vi "roboRIO v1.0 Close RSL.vi"(8 "error in (no error)":errorcluster, 10 "RSL Channel List":T3, 11 "myRIO Ref In":T1) -> (0 "error out":errorcluster)   [LabVIEW 2021]
uses:
  <vilib>/myRIO/Common/Instrument Driver Framework/roboRIO v1.0/RSL/typedefs/RSL Channels List.ctl
  <vilib>/myRIO/Common/Instrument Driver Framework/roboRIO v1.0/RSL/typedefs/RSL Channels Enum.ctl
  <vilib>/myRIO/Common/Instrument Driver Framework/Utilities/typedefs/myRIO v1.0 Reference.ctl
  <vilib>/myRIO/Common/Instrument Driver Framework/Utilities/typedefs/Generic FPGA Reference.ctl
  <vilib>/myRIO/Common/Instrument Driver Framework/roboRIO v1.0/RSL/vis/roboRIO v1.0 Build MUX Configuration RSL.vi
  <vilib>/myRIO/Common/Instrument Driver Framework/roboRIO v1.0/Resource Manager/vis/roboRIO v1.0 Unreserve Channel List.vi
  <vilib>/myRIO/Common/Instrument Driver Framework/roboRIO v1.0/Resource Manager/vis/roboRIO v1.0 Unreserve Channel.vi
  <vilib>/myRIO/Common/Instrument Driver Framework/roboRIO v1.0/Resource Manager/vis/roboRIO v1.0 Build Mutex Name.vi
  <vilib>/myRIO/Common/Instrument Driver Framework/Utilities/vis/Configuration Manager.vi
  <vilib>/myRIO/Common/Instrument Driver Framework/Utilities/vis/IO Manager.vi
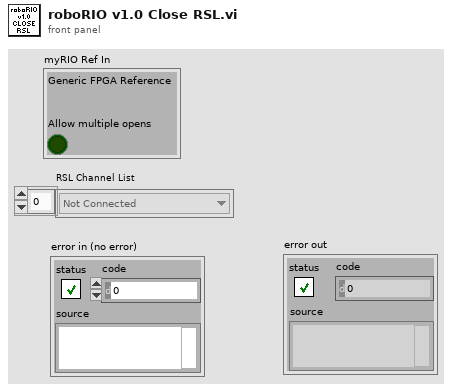
[diagram p1: front panel]
types:
  T1 = typedef "myRIO v1.0 Reference.ctl" = cluster{"Generic FPGA Reference":T2, "Allow multiple opens":bool}
  T2 = typedef "Generic FPGA Reference.ctl" = refnum<k20>
  T3 = typedef "RSL Channels List.ctl" = T4[]
  T4 = typedef "RSL Channels Enum.ctl" = enum16{"Not Connected", "RSL/RSL0"}
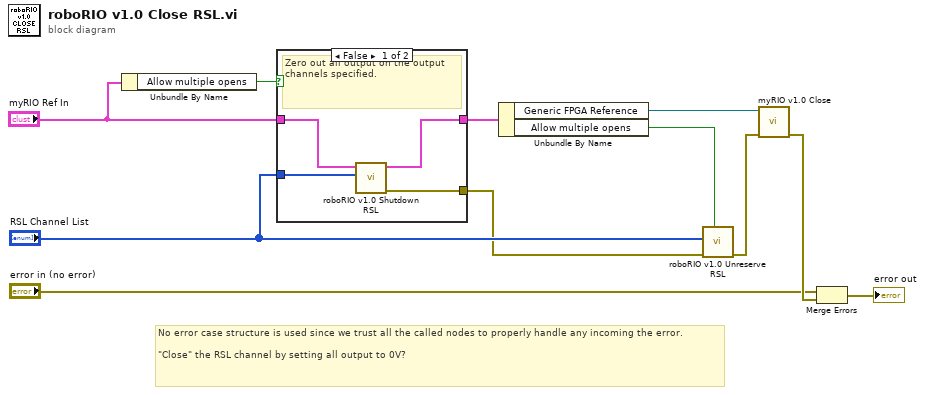
[diagram p0: block diagram]
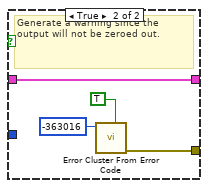
[diagram p2: hidden frame]
diagram:
  # "No error case structure is used since we trust all the called nodes to properly handle any incoming the error.\n\n\"Close\" the RSL channel by setting all output to 0V?"
  n1 = Unbundle By Name("myRIO Ref In") -> ("Allow multiple opens"=w6:bool)
  n2 = case shown="False" w6 {
    tunnel: "myRIO Ref In" -> [w15 w19]
    tunnel: [w14 w19] -> w8
    tunnel: "RSL Channel List" -> [w13 _]
    tunnel: [w12 w16] -> w2
    frame False {
      # "Zero out all output on the output channels specified."
      n3 = call <vilib>:"roboRIO v1.0 Shutdown RSL.vi"("Channel List"=w13, "myRIO Ref In"=w15) -> ("error out"=w12:errorcluster, "myRIO Ref Out"=w14:T1)  [unwired: 8 in]
    }
    frame True {
      # "Generate a warning since the output will not be zeroed out."
      n4 = call <vilib>:"Error Cluster From Error Code.vi"("is warning? (False)"=TRUE, "error code (0)"=-363016) -> ("error out"=w16:errorcluster)  [unwired: 7 in]
    }
  }
  n5 = Unbundle By Name(w8) -> ("Generic FPGA Reference"=w1:T2, "Allow multiple opens"=w9:bool)
  n6 = call <vilib>:"roboRIO v1.0 Unreserve RSL.vi"("Allow multiple opens?"=w9, "error in (no error)"=w2, "RSL Channel List"="RSL Channel List") -> ("error out"=w11:errorcluster)  [unwired: 8 in]
  n7 = call <vilib>:"myRIO v1.0 Close.vi"("error in (no error)"=w11, "myRIO FPGA Ref In"=w1) -> ("error out"=w10:errorcluster)  [unwired: 9 in]
  n8 = Merge Errors("error in (no error)", w10) -> (→"error out":errorcluster)
